vi "GetValueFromTreeControl.vi"(10 "ref in":refnum<vi>) -> (2 "데이터":string, 3 "ref out":refnum<vi>)   [LabVIEW 2018, in "Library-Ctrl.lvlib"]
uses:
  Library-Ctrl.lvlib
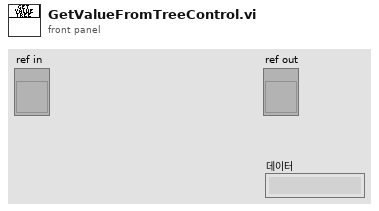
[diagram p1: front panel]
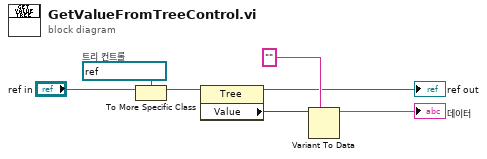
[diagram p0: block diagram]
diagram:
  w6 = refnum<vi> refnum  # 트리 컨트롤
  n1 = To More Specific Class(target class=w6, reference="ref in") -> (specific class reference=w5:refnum<vi>)  [unwired: 1 in, 1 out]
  n2 = property class="Tree"(reference=w5) -> (reference out=→"ref out":refnum<vi>, "Value"=w4:variant)  [unwired: 1 in, 1 out]
  n3 = Variant To Data(type="" ("값"), Variant=w4) -> (data=→"데이터":string)  [unwired: 1 in, 1 out]
